vi "SD_Keep_only_required_measurements.vi"(7 "byte order":T1(ring)=enum."little-endian", 8 "error in (no error)":errorcluster, 9 "Mode":bool, 10 "Variable":T5, 11 "Data in":T2 {"Measurements and statistics"."Running, perc. of time" format="%05.2f"}) -> (0 "error out":errorcluster, 1 "length, bytes":i32, 2 "Data string":string, 3 "Data out (copy)":T2 {"Measurements and statistics"."Running, perc. of time" format="%05.2f"})   [LabVIEW 2018, in "Stream Data.lvlib"]
uses:
  Stream Data.lvlib
  SubVi's/Controls/CTL_Full_data_frame.ctl
  SubVi's/Controls/CTL_Animal_Coordinates_and_Speed.ctl
  SubVi's/Controls/CTL_Measurements_and_Statistics.ctl
  Typedefs/CTL_Variable_to_pass.ctl
  Tracker.lvlib
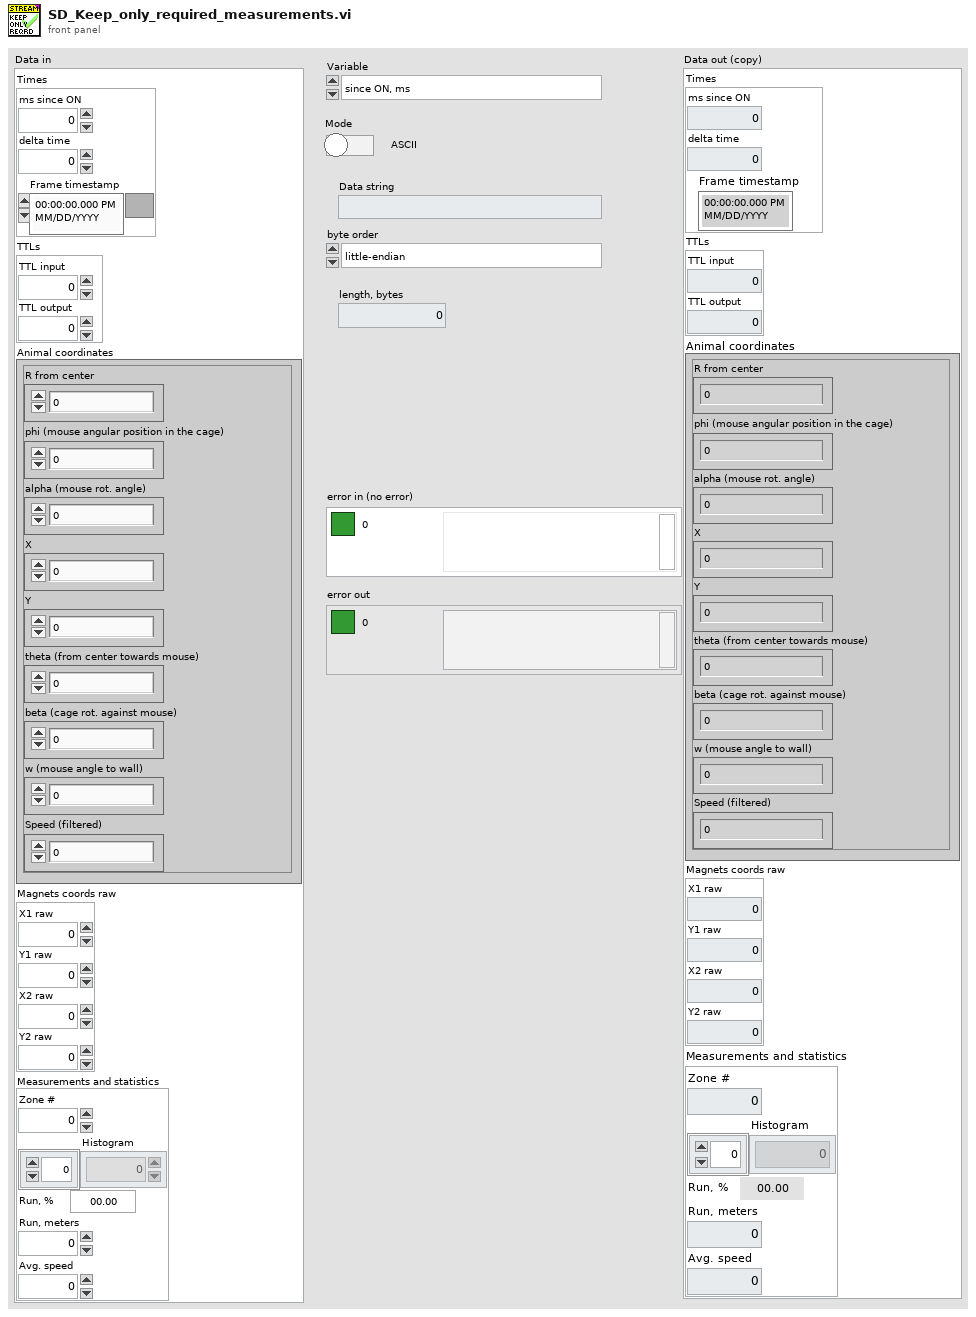
[diagram p1: front panel]
types:
  T1 = enum16{"big-endian, network order", "native, host order", "little-endian"}
  T2 = typedef "Tracker.lvlib/CTL_Full_data_frame.ctl" = cluster{"Times":cluster{"ms since ON":u32, "delta time":u32, "Frame timestamp":timestamp}, "TTLs":cluster{"TTL input":i16, "TTL output":i16}, "Animal coordinates":T3, "Magnets coords raw":cluster{"X1 raw":dbl, "Y1 raw":dbl, "X2 raw":dbl, "Y2 raw":dbl}, "Measurements and statistics":T4}
  T3 = typedef "Tracker.lvlib/CTL_Animal_Coordinates_and_Speed.ctl" = cluster{"R from center":dbl, "phi (mouse angular position in the cage)":dbl, "alpha (mouse rot. angle)":dbl, "X":dbl, "Y":dbl, "theta (from center towards mouse)":dbl, "beta (cage rot. against mouse)":dbl, "w (mouse angle to wall)":dbl, "Speed (filtered)":dbl}
  T4 = typedef "Tracker.lvlib/CTL_Measurements_and_Statistics.ctl" = cluster{"Zone #":i8, "Histogram":dbl[], "Running, perc. of time":dbl, "Run, meters":dbl, "Avg. speed":dbl}
  T5 = typedef "Stream Data.lvlib/CTL_Variable_to_pass.ctl" = enum16{"since ON, ms", "delta time, ms", "timestamp (SW)", "R", "phi", "alpha", "X", "Y", "Zone #", "Run percentage", "Speed, mm/s"}
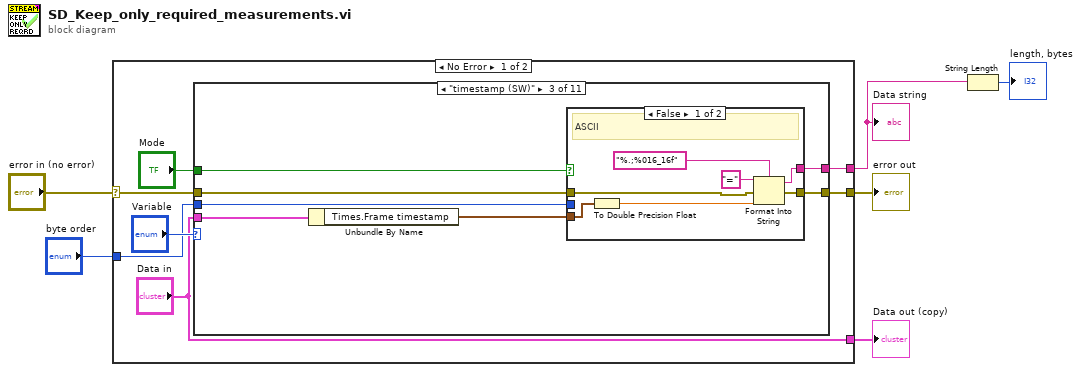
[diagram p0: block diagram]
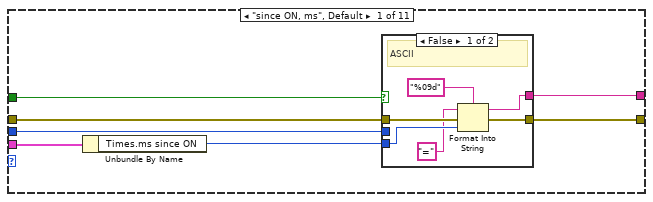
[diagram p2: hidden frame]
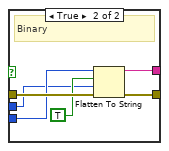
[diagram p3: hidden frame]
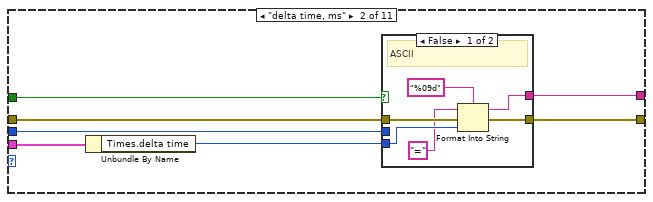
[diagram p4: hidden frame]
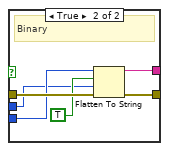
[diagram p5: hidden frame]
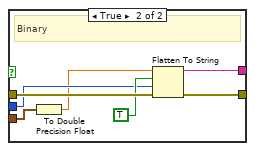
[diagram p6: hidden frame]
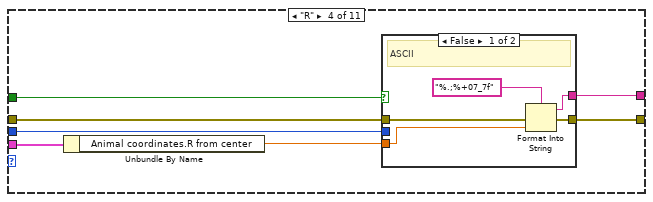
[diagram p7: hidden frame]
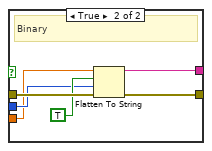
[diagram p8: hidden frame]
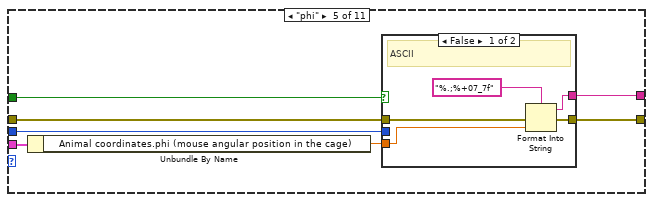
[diagram p9: hidden frame]
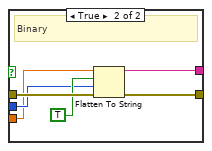
[diagram p10: hidden frame]
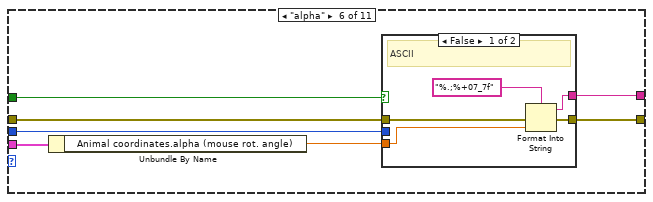
[diagram p11: hidden frame]
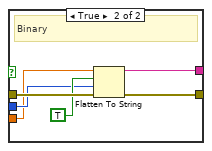
[diagram p12: hidden frame]
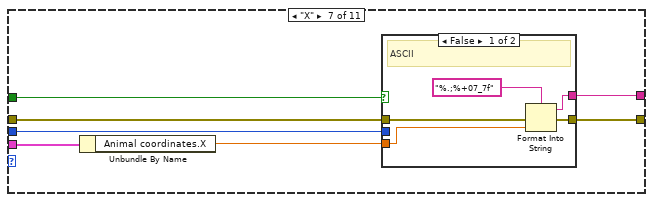
[diagram p13: hidden frame]
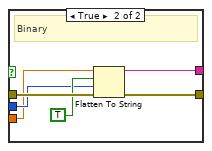
[diagram p14: hidden frame]
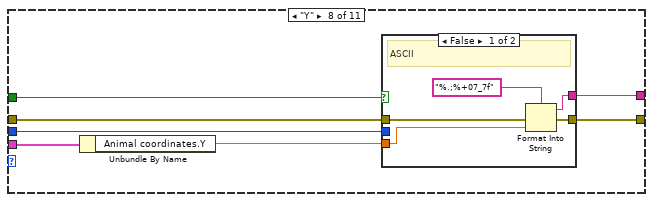
[diagram p15: hidden frame]
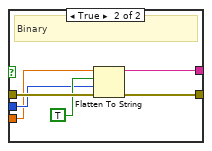
[diagram p16: hidden frame]
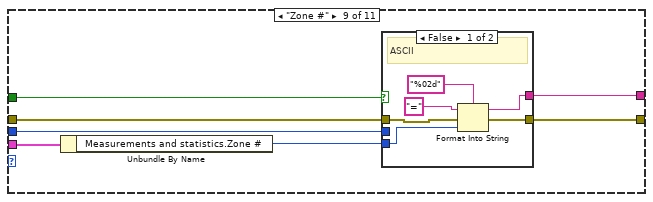
[diagram p17: hidden frame]
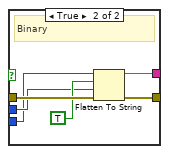
[diagram p18: hidden frame]
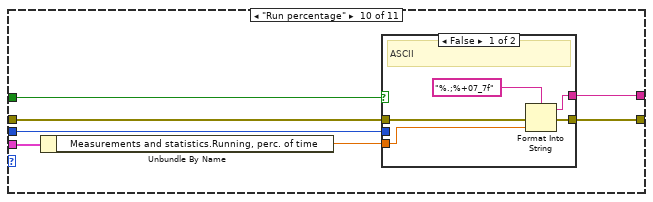
[diagram p19: hidden frame]
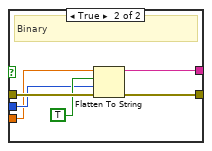
[diagram p20: hidden frame]
diagram:
  n1 = case shown="No Error" "error in (no error)" {
    selector: "error in (no error)" -> [w11 w218]
    tunnel: [w10 w218] -> w5
    tunnel: [w9 _] -> w1
    tunnel: ["Data in" _] -> w4
    tunnel: "byte order" -> [w7 _]
    frame No Error {
      n2 = case shown="\"timestamp (SW)\"" "Variable" {
        tunnel: "Data in" -> [w20 w39 w58 w79 w97 w115 w133 w151 w169 w188 w206]
        tunnel: "Mode" -> [w19 w38 w57 w78 w96 w114 w132 w150 w168 w187 w205]
        tunnel: [w17 w36 w55 w76 w94 w112 w130 w148 w166 w185 w203] -> w9
        tunnel: w11 -> [w16 w35 w54 w75 w93 w111 w129 w147 w165 w184 w202]
        tunnel: [w15 w34 w53 w74 w92 w110 w128 w146 w164 w183 w201] -> w10
        tunnel: w7 -> [w14 w33 w52 w73 w91 w109 w127 w145 w163 w182 w200]
        frame "since ON, ms", Default {
          n3 = Unbundle By Name(w20) -> ("Times.ms since ON"=w18:u32)
          n4 = case shown="False" w19 {
            tunnel: w18 -> [w26 w29]
            tunnel: [w24 w27] -> w17
            tunnel: w16 -> [w23 w32]
            tunnel: [w22 w31] -> w15
            tunnel: w14 -> [_ w28]
            frame False {
              # "ASCII"
              n5 = Format Into String(format string="%09d", initial string="=", error in=w23, w26) -> (resulting string=w24:string, error out=w22:errorcluster)
            }
            frame True {
              # "Binary"
              n6 = Flatten To String(anything=w29, prepend array or string size? (T)=TRUE, byte order (0:big-endian, network order)=w28, error in (no error)=w32) -> (data string=w27:string, error out=w31:errorcluster)  [unwired: 1 out]
            }
          }
        }
        frame "delta time, ms" {
          n7 = Unbundle By Name(w39) -> ("Times.delta time"=w37:u32)
          n8 = case shown="False" w38 {
            tunnel: w37 -> [w43 w48]
            tunnel: [w41 w46] -> w36
            tunnel: w35 -> [w44 w51]
            tunnel: [w42 w50] -> w34
            tunnel: w33 -> [_ w47]
            frame False {
              # "ASCII"
              n9 = Format Into String(format string="%09d", initial string="=", error in=w44, w43) -> (resulting string=w41:string, error out=w42:errorcluster)
            }
            frame True {
              # "Binary"
              n10 = Flatten To String(anything=w48, prepend array or string size? (T)=TRUE, byte order (0:big-endian, network order)=w47, error in (no error)=w51) -> (data string=w46:string, error out=w50:errorcluster)  [unwired: 1 out]
            }
          }
        }
        frame "timestamp (SW)" {
          n11 = Unbundle By Name(w58) -> ("Times.Frame timestamp"=w56:timestamp)
          n12 = case shown="False" w57 {
            tunnel: w56 -> [w61 w69]
            tunnel: [w62 w67] -> w55
            tunnel: w54 -> [w64 w72]
            tunnel: [w63 w71] -> w53
            tunnel: w52 -> [_ w68]
            frame False {
              # "ASCII"
              n13 = To Double Precision Float(number=w61) -> (double precision float=w60:dbl)
              n14 = Format Into String(format string="%.;%016_16f", initial string="=", error in=w64, w60) -> (resulting string=w62:string, error out=w63:errorcluster)
            }
            frame True {
              # "Binary"
              n15 = To Double Precision Float(number=w69) -> (double precision float=w66:dbl)
              n16 = Flatten To String(anything=w66, prepend array or string size? (T)=TRUE, byte order (0:big-endian, network order)=w68, error in (no error)=w72) -> (data string=w67:string, error out=w71:errorcluster)  [unwired: 1 out]
            }
          }
        }
        frame "R" {
          n17 = Unbundle By Name(w79) -> ("Animal coordinates.R from center"=w77:dbl)
          n18 = case shown="False" w78 {
            tunnel: w77 -> [w80 w85]
            tunnel: [w81 w86] -> w76
            tunnel: w75 -> [w83 w90]
            tunnel: [w82 w89] -> w74
            tunnel: w73 -> [_ w87]
            frame False {
              # "ASCII"
              n19 = Format Into String(format string="%.;%+07_7f", error in=w83, w80) -> (resulting string=w81:string, error out=w82:errorcluster)  [unwired: 1 in]
            }
            frame True {
              # "Binary"
              n20 = Flatten To String(anything=w85, prepend array or string size? (T)=TRUE, byte order (0:big-endian, network order)=w87, error in (no error)=w90) -> (data string=w86:string, error out=w89:errorcluster)  [unwired: 1 out]
            }
          }
        }
        frame "phi" {
          n21 = Unbundle By Name(w97) -> ("Animal coordinates.phi (mouse angular position in the cage)"=w95:dbl)
          n22 = case shown="False" w96 {
            tunnel: w95 -> [w100 w103]
            tunnel: [w98 w104] -> w94
            tunnel: w93 -> [w101 w108]
            tunnel: [w99 w107] -> w92
            tunnel: w91 -> [_ w105]
            frame False {
              # "ASCII"
              n23 = Format Into String(format string="%.;%+07_7f", error in=w101, w100) -> (resulting string=w98:string, error out=w99:errorcluster)  [unwired: 1 in]
            }
            frame True {
              # "Binary"
              n24 = Flatten To String(anything=w103, prepend array or string size? (T)=TRUE, byte order (0:big-endian, network order)=w105, error in (no error)=w108) -> (data string=w104:string, error out=w107:errorcluster)  [unwired: 1 out]
            }
          }
        }
        frame "alpha" {
          n25 = Unbundle By Name(w115) -> ("Animal coordinates.alpha (mouse rot. angle)"=w113:dbl)
          n26 = case shown="False" w114 {
            tunnel: w113 -> [w117 w121]
            tunnel: [w116 w122] -> w112
            tunnel: w111 -> [w119 w126]
            tunnel: [w118 w125] -> w110
            tunnel: w109 -> [_ w123]
            frame False {
              # "ASCII"
              n27 = Format Into String(format string="%.;%+07_7f", error in=w119, w117) -> (resulting string=w116:string, error out=w118:errorcluster)  [unwired: 1 in]
            }
            frame True {
              # "Binary"
              n28 = Flatten To String(anything=w121, prepend array or string size? (T)=TRUE, byte order (0:big-endian, network order)=w123, error in (no error)=w126) -> (data string=w122:string, error out=w125:errorcluster)  [unwired: 1 out]
            }
          }
        }
        frame "X" {
          n29 = Unbundle By Name(w133) -> ("Animal coordinates.X"=w131:dbl)
          n30 = case shown="False" w132 {
            tunnel: w131 -> [w134 w139]
            tunnel: [w135 w140] -> w130
            tunnel: w129 -> [w137 w144]
            tunnel: [w136 w143] -> w128
            tunnel: w127 -> [_ w141]
            frame False {
              # "ASCII"
              n31 = Format Into String(format string="%.;%+07_7f", error in=w137, w134) -> (resulting string=w135:string, error out=w136:errorcluster)  [unwired: 1 in]
            }
            frame True {
              # "Binary"
              n32 = Flatten To String(anything=w139, prepend array or string size? (T)=TRUE, byte order (0:big-endian, network order)=w141, error in (no error)=w144) -> (data string=w140:string, error out=w143:errorcluster)  [unwired: 1 out]
            }
          }
        }
        frame "Y" {
          n33 = Unbundle By Name(w151) -> ("Animal coordinates.Y"=w149:dbl)
          n34 = case shown="False" w150 {
            tunnel: w149 -> [w152 w157]
            tunnel: [w153 w158] -> w148
            tunnel: w147 -> [w155 w162]
            tunnel: [w154 w161] -> w146
            tunnel: w145 -> [_ w159]
            frame False {
              # "ASCII"
              n35 = Format Into String(format string="%.;%+07_7f", error in=w155, w152) -> (resulting string=w153:string, error out=w154:errorcluster)  [unwired: 1 in]
            }
            frame True {
              # "Binary"
              n36 = Flatten To String(anything=w157, prepend array or string size? (T)=TRUE, byte order (0:big-endian, network order)=w159, error in (no error)=w162) -> (data string=w158:string, error out=w161:errorcluster)  [unwired: 1 out]
            }
          }
        }
        frame "Zone #" {
          n37 = Unbundle By Name(w169) -> ("Measurements and statistics.Zone #"=w167:i8)
          n38 = case shown="False" w168 {
            tunnel: w167 -> [w171 w176]
            tunnel: [w172 w177] -> w166
            tunnel: w165 -> [w174 w181]
            tunnel: [w173 w180] -> w164
            tunnel: w163 -> [_ w178]
            frame False {
              # "ASCII"
              n39 = Format Into String(format string="%02d", initial string="=", error in=w174, w171) -> (resulting string=w172:string, error out=w173:errorcluster)
            }
            frame True {
              # "Binary"
              n40 = Flatten To String(anything=w176, prepend array or string size? (T)=TRUE, byte order (0:big-endian, network order)=w178, error in (no error)=w181) -> (data string=w177:string, error out=w180:errorcluster)  [unwired: 1 out]
            }
          }
        }
        frame "Run percentage" {
          n41 = Unbundle By Name(w188) -> ("Measurements and statistics.Running, perc. of time"=w186:dbl)
          n42 = case shown="False" w187 {
            tunnel: w186 -> [w189 w194]
            tunnel: [w190 w195] -> w185
            tunnel: w184 -> [w192 w199]
            tunnel: [w191 w198] -> w183
            tunnel: w182 -> [_ w196]
            frame False {
              # "ASCII"
              n43 = Format Into String(format string="%.;%+07_7f", error in=w192, w189) -> (resulting string=w190:string, error out=w191:errorcluster)  [unwired: 1 in]
            }
            frame True {
              # "Binary"
              n44 = Flatten To String(anything=w194, prepend array or string size? (T)=TRUE, byte order (0:big-endian, network order)=w196, error in (no error)=w199) -> (data string=w195:string, error out=w198:errorcluster)  [unwired: 1 out]
            }
          }
        }
        frame "Speed, mm/s" {
          n45 = Unbundle By Name(w206) -> ("Animal coordinates.Speed (filtered)"=w204:dbl)
          n46 = case shown="False" w205 {
            tunnel: w204 -> [w207 w212]
            tunnel: [w208 w213] -> w203
            tunnel: w202 -> [w210 w217]
            tunnel: [w209 w216] -> w201
            tunnel: w200 -> [_ w214]
            frame False {
              # "ASCII"
              n47 = Format Into String(format string="%.;%+07_7f", error in=w210, w207) -> (resulting string=w208:string, error out=w209:errorcluster)  [unwired: 1 in]
            }
            frame True {
              # "Binary"
              n48 = Flatten To String(anything=w212, prepend array or string size? (T)=TRUE, byte order (0:big-endian, network order)=w214, error in (no error)=w217) -> (data string=w213:string, error out=w216:errorcluster)  [unwired: 1 out]
            }
          }
        }
      }
    }
    frame Error {
    }
  }
  "error out" <- w5
  "Data string" <- w1
  "Data out (copy)" <- w4
  n49 = String Length(string=w1) -> (length=→"length, bytes":i32)
